vi "NIDCPower_channel_ganging - measure multiple.vi"(8 "error in (no error)":errorcluster, 9 "timeout (1.0)":dbl=1.0 format="%.6p", 10 "count (1)":i32=1, 11 "Ganged Session In":T1) -> (0 "error out":errorcluster, 1 "current measurements":dbl[](array[numeric]) caption="channel current measurements", 2 "voltage measurements":dbl[](array[numeric]), 3 "Ganged Session Out":T1, 4 "Some Channels in compliance?":bool, 5 "ganged current measurement":dbl, 6 "All Channels in compliance?":bool, 7 "ganged voltage measurement":dbl)   [LabVIEW 2021]
uses:
  ctl/NIDCPower_channel_ganging - ctl - ganged session.ctl
  ctl/NIDCPower_channel_ganging - ctl - ganged config.ctl
  ctl/NIDCPower_channel_ganging - ctl - channel mode.ctl
  <vilib>/Analysis/baseanly.llb/Mean (DBL).vi
  <vilib>/Analysis/NI_AALBase.lvlib
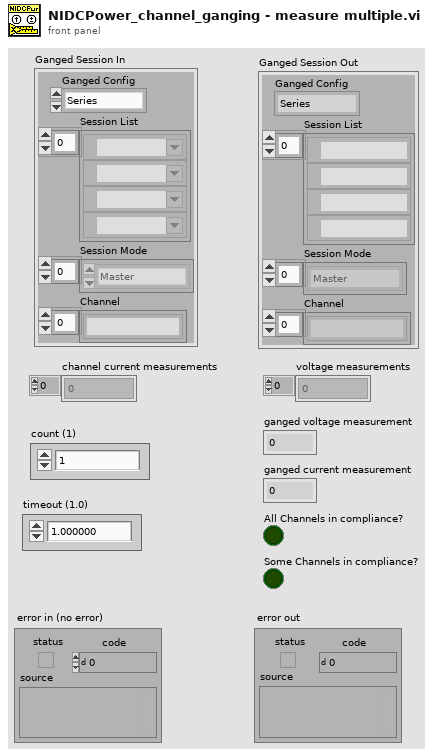
[diagram p1: front panel]
types:
  T1 = typedef "NIDCPower_channel_ganging - ctl - ganged session.ctl" = cluster{"Ganged Config":T2, "Session List":refnum<k15>[], "Session Mode":T3[], "Channel":string[]}
  T2 = typedef "NIDCPower_channel_ganging - ctl - ganged config.ctl" = enum32{"Series", "Parallel", "Manual"}
  T3 = typedef "NIDCPower_channel_ganging - ctl - channel mode.ctl" = enum32{"Master", "Slave", "Slave - Inverted"}
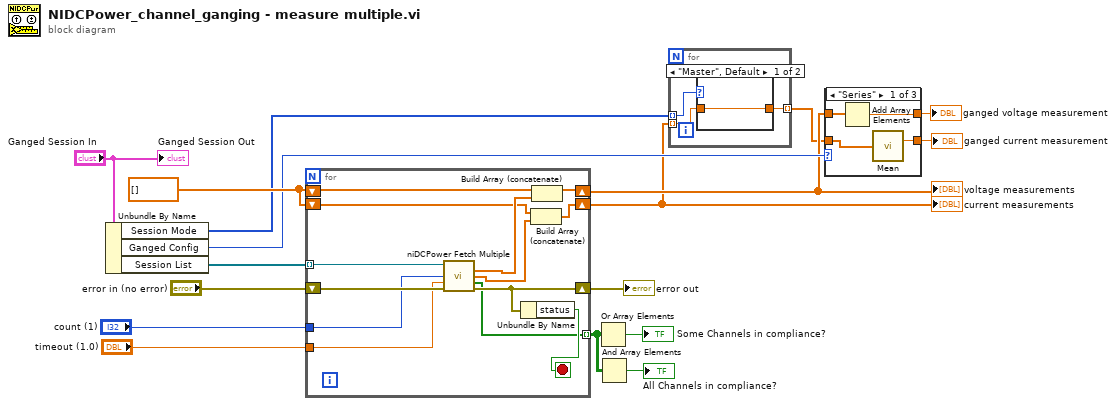
[diagram p0: block diagram]
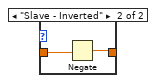
[diagram p2: hidden frame]
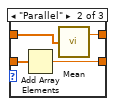
[diagram p3: hidden frame]
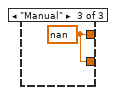
[diagram p4: hidden frame]
diagram:
  w15 = dbl[] [] ("voltage measurements")
  n1 = Unbundle By Name("Ganged Session In") -> ("Session Mode"=w3:T3[], "Ganged Config"=w11:T2, "Session List"=w13:refnum<k15>[])
  n2 = for {
    shift-right: [w22] -> w16
    shift-left: "error in (no error)" -> [w30]
    tunnel: w13 -> [w29] mode=indexing
    shift-right: [w26] -> w10
    shift-left: w15 -> [w28]
    shift-right: [w23] -> w5
    shift-left: w15 -> [w25]
    tunnel: [w20] -> w6 mode=indexing
    tunnel: "count (1)" -> [w19]
    tunnel: "timeout (1.0)" -> [w18]
    stop <- w21 stop-if-true
    n3 = call <instrlib>:"niDCPower Fetch Multiple.vi"("instrument handle"=w29, "count (1)"=w19, "timeout (1.0)"=w18, "error in (no error)"=w30) -> ("voltage measurements"=w27:dbl[], "current measurements"=w24:dbl[], "in compliance"=w20:bool[], "error out"=w22:errorcluster)  [unwired: 6 in, 2 out]
    n4 = Unbundle By Name(w22) -> ("status"=w21:bool)
    n5 = Build Array (concatenate)(w25, w24) -> (w23:dbl[])
    n6 = Build Array (concatenate)(w28, w27) -> (w26:dbl[])
  }
  "error out" <- w16
  "voltage measurements" <- w10
  "current measurements" <- w5
  n7 = Or Array Elements(Boolean array=w6) -> (logical OR=→"Some Channels in compliance?":bool)
  n8 = And Array Elements(Boolean array=w6) -> (logical AND=→"All Channels in compliance?":bool)
  n9 = for {
    tunnel: w3 -> [w33] mode=indexing
    tunnel: w5 -> [w32] mode=indexing
    tunnel: [w31] -> w4 mode=indexing
    n10 = case shown="\"Master\", Default" w33 {
      tunnel: [w34 w36] -> w31
      tunnel: w32 -> [w34 w35]
      frame "Master", Default {
      }
      frame "Slave - Inverted" {
        n11 = Negate(x=w35) -> (-x=w36:dbl)
      }
    }
  }
  n12 = case shown="\"Series\"" w11 {
    tunnel: w10 -> [w40 w42 _]
    tunnel: w4 -> [w38 w44 _]
    tunnel: [w37 w43 w45] -> w8
    tunnel: [w39 w41 w45] -> w9
    frame "Series" {
      n13 = Add Array Elements(numeric array=w40) -> (sum=w39:dbl)
      n14 = call-poly <vilib>:"Mean.vi"("X"=w38) -> ("mean"=w37:dbl)  [unwired: 1 out]
    }
    frame "Parallel" {
      n15 = Add Array Elements(numeric array=w44) -> (sum=w43:dbl)
      n16 = call-poly <vilib>:"Mean.vi"("X"=w42) -> ("mean"=w41:dbl)  [unwired: 1 out]
    }
    frame "Manual" {
      w45 = nan
    }
  }
  "ganged voltage measurement" <- w9
  "ganged current measurement" <- w8
  "Ganged Session Out" <- "Ganged Session In"
